vi "Set AF Software Limits.vi"(0 "VISA Resource Name":refnum<visa-resource-name>, 5 "Device Number (1)":i32=1, 7 "Near Limit (30000.0 um)":dbl=30000.0 format="%.1f", 9 "Far Limit (0.01 um)":dbl=0.01, 11 "error in (no error)":errorcluster {"code" format="%.0x"}) -> (4 "VISA Resource Name Out":refnum<visa-resource-name>, 15 "error out":errorcluster {"code" format="%.0x"})   [LabVIEW 2020, in "Olympus IX BX Series.lvlib"]
doc: "Sets the software limits of the AF control range."
uses:
  Olympus IX BX Series.lvlib
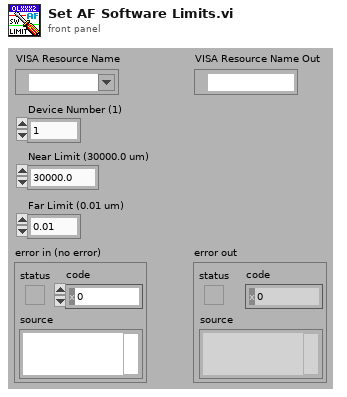
[diagram p1: front panel]
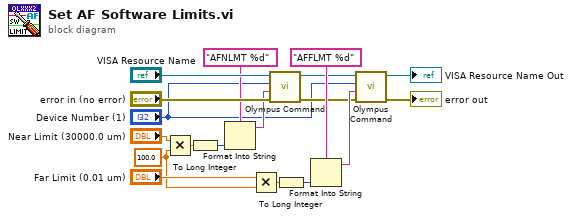
[diagram p0: block diagram]
diagram:
  w2 = 100.0 ("y")
  n1 = Multiply(x="Near Limit (30000.0 um)", y=w2) -> (x*y=w18:dbl)
  n2 = To Long Integer(number=w18) -> (32bit integer=w12:i32)
  n3 = Format Into String(format string="AFNLMT %d", w12) -> (resulting string=w15:string)  [unwired: 2 in, 1 out]
  n4 = Multiply(x="Far Limit (0.01 um)", y=w2) -> (x*y=w11:dbl)
  n5 = call "Olympus Command.vi"("error in (no error)"="error in (no error)", "Command string"=w15, "Device Number (1)"="Device Number (1)", "VISA Resource Name"="VISA Resource Name") -> ("error out"=w5:errorcluster, "VISA Resource Name Out"=w4:refnum<visa-resource-name>)  [unwired: 5 in, 1 out]
  n6 = To Long Integer(number=w11) -> (32bit integer=w8:i32)
  n7 = Format Into String(format string="AFFLMT %d", w8) -> (resulting string=w10:string)  [unwired: 2 in, 1 out]
  n8 = call "Olympus Command.vi"("error in (no error)"=w5, "Command string"=w10, "Device Number (1)"="Device Number (1)", "VISA Resource Name"=w4) -> ("error out"=→"error out":errorcluster, "VISA Resource Name Out"=→"VISA Resource Name Out":refnum<visa-resource-name>)  [unwired: 5 in, 1 out]
